vi "Run Inject.vi"(6 "Wait for pump":bool, 7 "auto_switch_valve":bool=TRUE, 8 "error in (no error)":errorcluster, 11 "PHD Ultra in":refnum<class "cetoni.lvclass">) -> (0 "error out":errorcluster, 3 "PHD Ultra out":refnum<class "cetoni.lvclass">)   [LabVIEW 2018, in "cetoni.lvlib" / "cetoni.lvclass"]
uses:
  cetoni.lvclass
  Resources/GLOBAL/GLOBAL Time-critical.vi
  <userlib>/QmixLib/QmixLib.lvlib
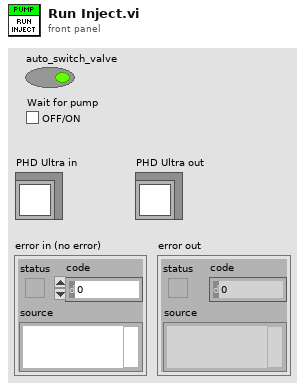
[diagram p1: front panel]
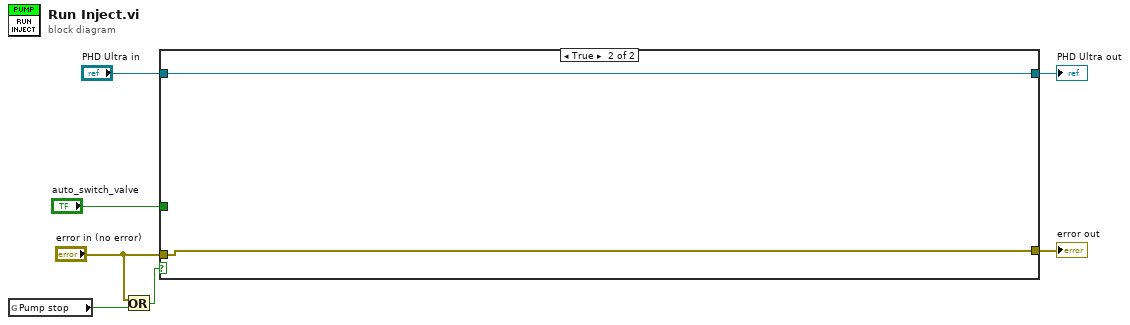
[diagram p0: block diagram]
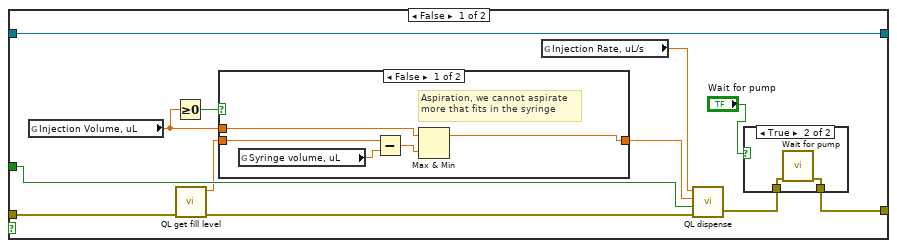
[diagram p2: hidden frame]
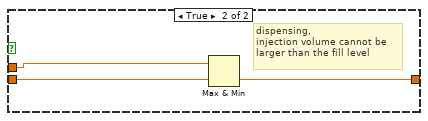
[diagram p4: hidden frame]
diagram:
  n1 = global read "GLOBAL Time-critical.vi" "Pump stop"() -> (w3:bool)
  n2 = Or(x="error in (no error)", y=w3) -> (x .or. y?=w2:bool)
  n3 = case shown="True" w2 {
    tunnel: [w10 w31] -> w7
    tunnel: [w18 w32] -> w5
    tunnel: "PHD Ultra in" -> [w18 w32]
    tunnel: "auto_switch_valve" -> [w19 _]
    tunnel: "error in (no error)" -> [w8 w31]
    frame False {
      n4 = global read "GLOBAL Time-critical.vi" "Injection Volume, uL"() -> (w15:dbl)
      n5 = Greater Or Equal To 0?(x=w15) -> (x >= 0?=w16:bool)
      n6 = call <userlib>:"QL get fill level.vi"("error in (no error)"=w8) -> ("error out"=w12:errorcluster, "Fill level, uL"=w14:dbl)  [unwired: 9 in]
      n7 = case shown="False" w16 {
        tunnel: w15 -> [w24 w30]
        tunnel: w14 -> [w25 w29]
        tunnel: [w23 w28] -> w13
        frame False {
          # "Aspiration, we cannot aspirate\nmore that fits in the syringe"
          n8 = global read "GLOBAL Time-critical.vi" "Syringe volume, uL"() -> (w27:dbl)
          n9 = Subtract(x=w25, y=w27) -> (x-y=w26:dbl)
          n10 = Max & Min(x=w24, y=w26) -> (max(x,y)=w23:dbl)  [unwired: 1 out]
        }
        frame True {
          # "dispensing,\ninjection volume cannot be\nlarger than the fill level"
          n11 = Max & Min(x=w30, y=w29) -> (min(x,y)=w28:dbl)  [unwired: 1 out]
        }
      }
      n12 = global read "GLOBAL Time-critical.vi" "Injection Rate, uL/s"() -> (w17:dbl)
      n13 = call <userlib>:"QL dispense.vi"("error in (no error)"=w12, "auto_switch_valve"=w19, "volume_uL"=w13, "flow_rate_uL_s"=w17) -> ("error out"=w11:errorcluster)  [unwired: 3 in]
      n14 = case shown="True" "Wait for pump" {
        tunnel: w11 -> [w20 w22]
        tunnel: [w20 w21] -> w10
        frame False {
        }
        frame True {
          n15 = call "Wait for pump.vi"("error in (no error)"=w22) -> ("error out"=w21:errorcluster)  [unwired: 10 in]
        }
      }
    }
    frame True {
    }
  }
  "error out" <- w7
  "PHD Ultra out" <- w5
